vi "AwakeRunnerNoScreen.vi"() -> ()   [LabVIEW 2011]
uses:
  <vilib>/vision/Image Controls.llb/IMAQ Image.ctl
  <vilib>/Instr/_visa.llb/Select Event Type.ctl
  <instrlib>/niHWS/nihws.llb/niHWS Open File Permissions ID.ctl
  <vilib>/DAQmx/read.llb/DAQmx Read (Analog Wfm 1Chan NSamp).vi
  <instrlib>/niHWS/nihws.llb/niHWS Write Analog DBL.vi
  <instrlib>/niHWS/nihws.llb/niHWS Write Analog WDT.vi
  <vilib>/DAQmx/miscellaneous.llb/DAQmx Fill In Error Info.vi
  <vilib>/express/express arith-compare/Formula/XNode/ExpressFormulaBlockNode.xnode
  C:/Program Files/National Instruments/LabVIEW 2011/resource/objmgr/daqmx.rc
  <vilib>/vision/NI_Vision_Development_Module.lvlib
  <vilib>/ptbypt/NI_PtbyPt.lvlib
panel:
  out "Click Value":i8
  out "Image Dst Out":T1
  out "Ephys Rate":dbl=1000.0
  out "Waveform Chart":waveform(dbl)(graph)
  out "Speed History":dbl(graph)
  in  "Magnify":bool
  in  "stop":bool
  out "Camera":T1(plugin-control)
  out "Rec Time":dbl format="%#_3g"
  out "fps":dbl format="%#_2g"
  in  "Rec":bool
  in  "Path":path
  in  "Gain":dbl(slide)=2.6607250597988097 min=1.0 max=3.9810717055349722 scale=0.0..4.0
  in  "Exposure Time":dbl(slide)=16602.0 min=56.0 max=16602.0 scale=0.0..16600.0
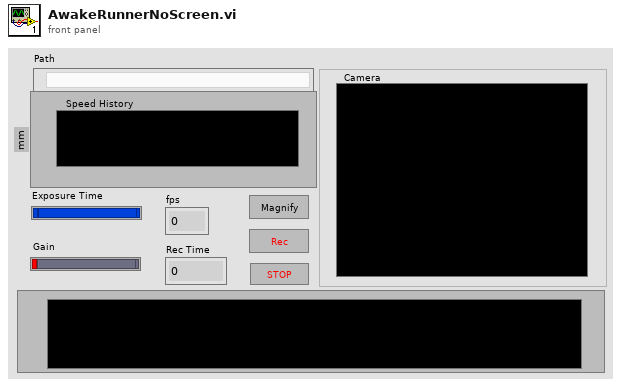
[diagram p1: front panel]
types:
  T1 = typedef "IMAQ Image.ctl" = refnum<image>
  T2 = enum32{"Invalid", "Standard", "Closed", "Hidden", "Minimized", "Maximized"}
  T3 = typedef "niHWS Open File Permissions ID.ctl" = enum32{"Read Only", "Read/Write Existing", "Read/Write/Create New", "Read/Write/Create New Always"}
  T4 = typedef "AviRefnum.ctl" = refnum<k1>
  T5 = typedef "Select Event Type.ctl" = u32
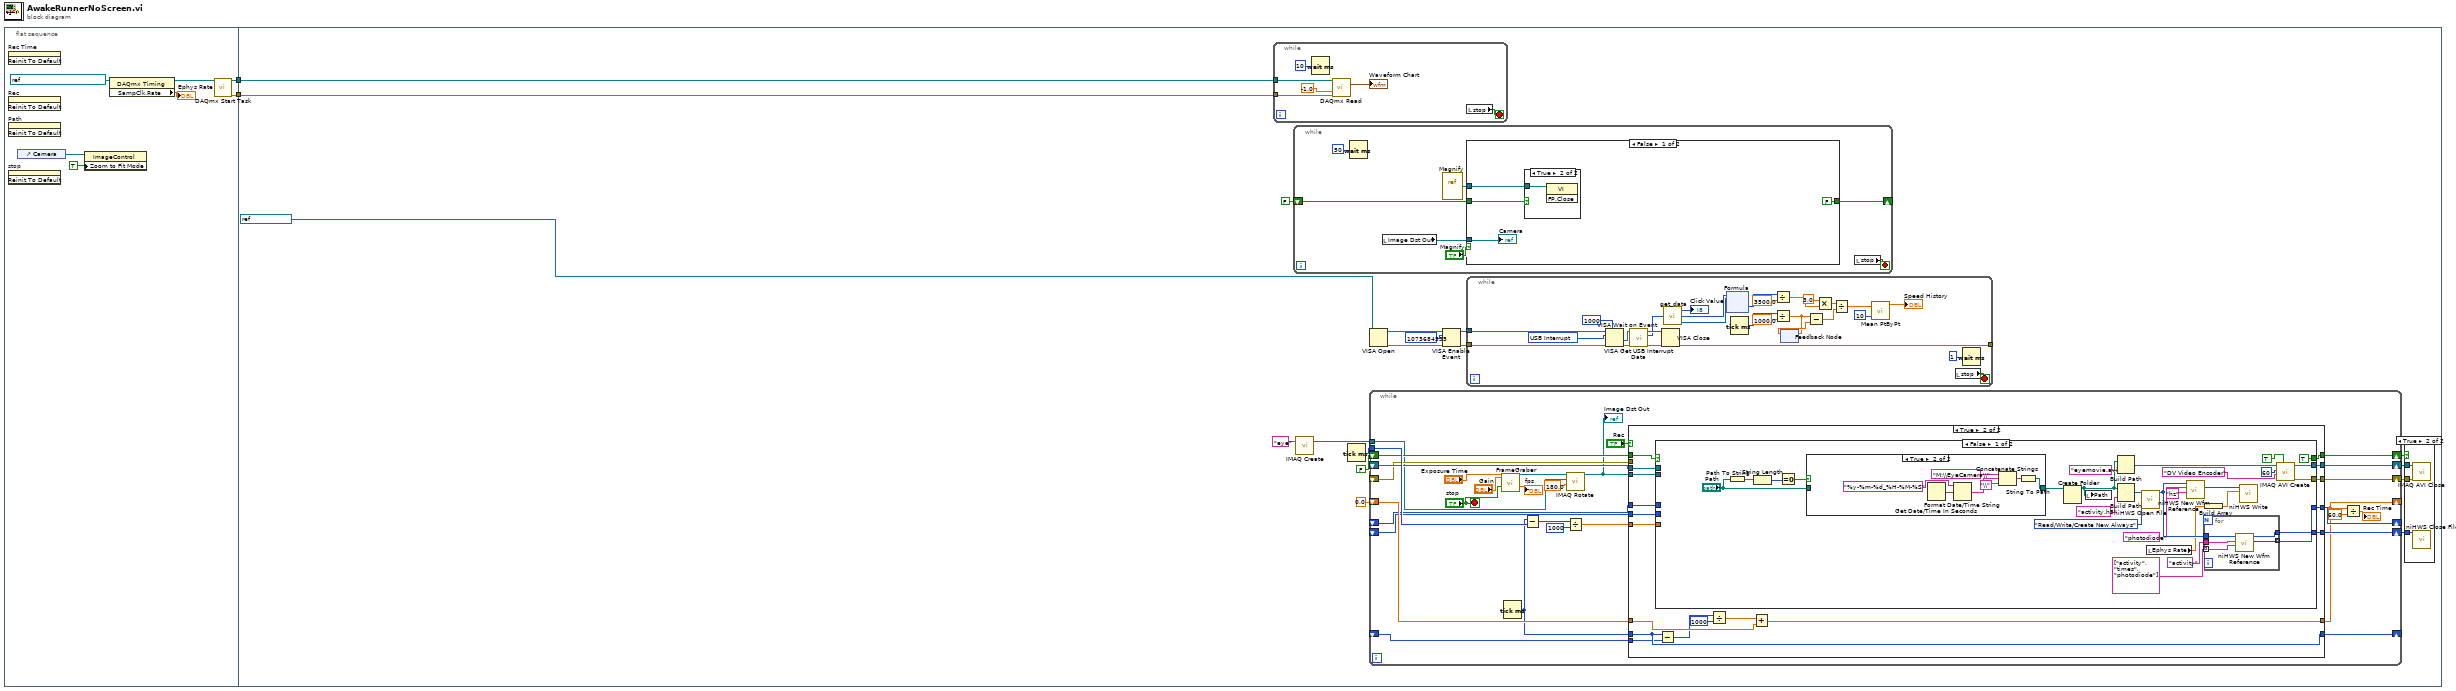
[diagram p0: block diagram]
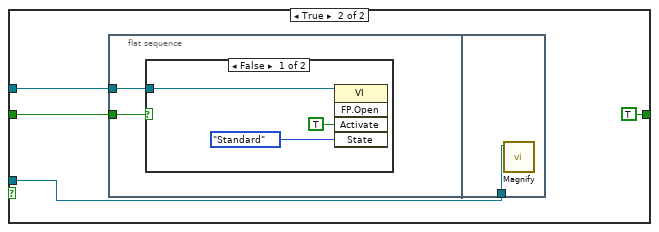
[diagram p3: hidden frame]
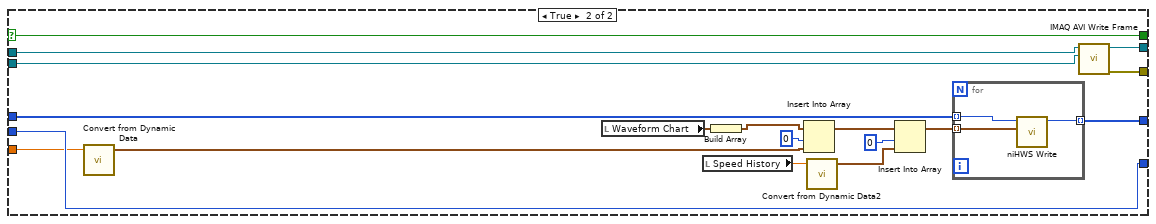
[diagram p8: hidden frame]
diagram:
  n1 = flat-sequence {
    tunnel: [w7] -> w2
    tunnel: [w6] -> w1
    tunnel: w2 -> [w19]
    tunnel: w1 -> [w18]
    frame #0 {
      n2 = invoke on="Rec Time" class="DigNum (strict)" method="Reinit To Default"() -> ()  [unwired: 3 in, 3 out]
      n3 = invoke on="Rec" class="Bool (strict)" method="Reinit To Default"() -> ()  [unwired: 3 in, 3 out]
      n4 = invoke on="Path" class="Path" method="Reinit To Default"() -> ()  [unwired: 3 in, 3 out]
      n5 = invoke on="stop" class="Bool (strict)" method="Reinit To Default"() -> ()  [unwired: 3 in, 3 out]
      n6 = control-ref of="Camera"() -> (w9:refnum<vi>)
      n7 = property on="Property Node" class="ImageControl"(reference=w9, "Zoom to Fit Mode"=TRUE) -> ()  [unwired: 1 in, 2 out]
      n8 = property class="DAQmx Timing"(reference=refnum<k21> "Photodiode Intrinsic Imaging" ("task/channels in")) -> (reference out=w3:refnum<k21>, "SampClk.Rate"=→"Ephys Rate":dbl)  [unwired: 1 in, 1 out]
      n9 = call <vilib>:"DAQmx Start Task.vi"("task/channels in"=w3) -> ("task out"=w7:refnum<k21>, "error out"=w6:errorcluster)  [unwired: 13 in]
    }
    frame #1 {
      n10 = while {
        tunnel: w19 -> [w70]
        tunnel: w18 -> [w69]
        stop <- w71 stop-if-true
        n11 = Wait (ms)(milliseconds to wait=u32 10) -> ()  [unwired: 1 out]
        n12 = call-poly <vilib>:"DAQmx Read.vi"("task/channels in"=w70, "timeout"=-1.0, "error in"=w69) -> ("data"=→"Waveform Chart":waveform(dbl))  [unwired: 10 in, 2 out]
        n13 = local read "stop"() -> (w71:bool)
      }
      n14 = while {
        shift-right: [w75] -> _
        shift-left: FALSE -> [w74]
        stop <- w76 stop-if-true
        n15 = Wait (ms)(milliseconds to wait=u32 50) -> ()  [unwired: 1 out]
        n16 = local read "Image Dst Out"() -> (w72:T1)
        n17 = vi-ref "Magnify.vi"() -> (w78:refnum<vi>)
        n18 = case shown="False" "Magnify" {
          tunnel: w78 -> [w82 w87]
          tunnel: [FALSE TRUE] -> w75
          tunnel: w74 -> [w81 w85]
          tunnel: w72 -> [w79 w84]
          frame False {
            n19 = case shown="True" w81 {
              tunnel: w82 -> [_ w83]
              frame False {
              }
              frame True {
                n20 = invoke class="VI" method="FP.Close"(reference=w83) -> ()  [unwired: 2 in, 3 out]
              }
            }
            "Camera" <- w79
          }
          frame True {
            n21 = flat-sequence {
              tunnel: w87 -> [w89]
              tunnel: w85 -> [w88]
              tunnel: w84 -> [w93]
              frame #0 {
                n22 = case shown="False" w88 {
                  tunnel: w89 -> [w91 _]
                  frame False {
                    n23 = invoke class="VI" method="FP.Open"(reference=w91, "Activate"=TRUE ("Wait Until Done"), "State"=T2."Standard") -> ()  [unwired: 2 in, 5 out]
                  }
                  frame True {
                  }
                }
              }
              frame #1 {
                n24 = call "Magnify.vi"("Camera 2"=w93) -> ()  [unwired: 11 in]
              }
            }
          }
        }
        n25 = local read "stop"() -> (w76:bool)
      }
      n26 = call "IMAQ Create"("Image Name"="eye") -> ("New Image"=w10:T1)  [unwired: 4 in, 1 out]
      n27 = Tick Count (ms)() -> (millisecond timer value=w24:u32)
      n28 = VISA Open(VISA resource name=refnum<visa-resource-name> "Mouse") -> (VISA resource name=w14:refnum<visa-resource-name>, error out=w13:errorcluster)  [unwired: 1 in, 3 out]
      n29 = while {
        tunnel: w24 -> [w125]
        shift-right: [w124] -> _
        shift-left: _ -> [w123]
        shift-right: [w104] -> _
        shift-left: 0.0 -> [w122]
        shift-right: [w112] -> w22
        shift-left: FALSE -> [w113]
        shift-right: [w109] -> _
        shift-left: _ -> [w108]
        shift-right: [w110] -> w21
        shift-left: _ -> [w107]
        shift-right: [w126] -> w27
        shift-left: _ -> [w106]
        shift-right: [w97] -> w26
        shift-left: _ -> [w105]
        tunnel: w10 -> [w98]
        stop <- "stop" stop-if-true
        n30 = call "FrameGraber.vi"("Exposure Time"="Exposure Time", "Gain"="Gain", "Stop (F)"="stop") -> ("Image Out"=w101:T1, "Frame Rate"=→"fps":dbl)  [unwired: 20 in, 3 out]
        n31 = Tick Count (ms)() -> (millisecond timer value=w114:u32)
        n32 = Subtract(x=w114, y=w125) -> (x-y=w117:u32)
        n33 = call "IMAQ Rotate"("Angle (degrees)"=sgl 180.0, "Image Dst"=w98, "Image Src"=w101) -> ("Image Dst Out"=w100:T1)  [unwired: 7 in, 1 out]
        "Image Dst Out" <- w100
        n34 = Divide(x=w117, y=1000) -> (x/y=w115:dbl)
        n35 = case shown="True" "Rec" {
          tunnel: [w128 w142] -> w126
          tunnel: [w127 w141] -> w97
          tunnel: [w132 w148] -> w104
          tunnel: w115 -> [_ w139]
          tunnel: [w133 w151] -> w124
          tunnel: w114 -> [w133 w151]
          tunnel: w123 -> [_ w150]
          tunnel: w122 -> [w132 w149]
          tunnel: w100 -> [_ w140]
          tunnel: w113 -> [w131 w144]
          tunnel: [w131 w143] -> w112
          tunnel: [w129 w138] -> w110
          tunnel: [w130 w137] -> w109
          tunnel: w108 -> [w130 w136]
          tunnel: w107 -> [w129 w135]
          tunnel: w106 -> [w128 w134]
          tunnel: w105 -> [w127 _]
          frame False {
          }
          frame True {
            n36 = case shown="False" w144 {
              selector: w144 -> [_ w209]
              tunnel: [TRUE w209] -> w143
              tunnel: [w175 w208] -> w142
              tunnel: [w174 w207] -> w141
              tunnel: w140 -> [_ w206]
              tunnel: w139 -> [_ w202]
              tunnel: [w159 w205] -> w138
              tunnel: [w158 w194] -> w137
              tunnel: w136 -> [_ w195]
              tunnel: w135 -> [_ w205]
              tunnel: w134 -> [_ w204]
              frame False {
                n37 = Path To String(path="Path") -> (string=w176:string)
                n38 = String Length(string=w176) -> (length=w177:i32)
                n39 = Equal To 0?(x=w177) -> (x = 0?=w165:bool)
                n40 = case shown="True" w165 {
                  tunnel: [w184 w185] -> w163
                  tunnel: "Path" -> [w184 _]
                  frame False {
                  }
                  frame True {
                    n41 = Get Date/Time In Seconds() -> (seconds since 1Jan1904=w191:timestamp)
                    n42 = Format Date/Time String(time format string (%c)="%y-%m-%d_%H-%M-%S", seconds (now)=w191) -> (date/time string=w188:string)  [unwired: 1 in]
                    n43 = Concatenate Strings("M:\\EyeCamera\\", w188, "\\" ("string")) -> (w186:string)
                    n44 = String To Path(string=w186) -> (path=w185:path)
                  }
                }
                n45 = Create Folder(path (use dialog)=w163) -> (created path=w162:path)  [unwired: 2 in, 2 out]
                n46 = local write "Path"(w162) -> ()
                n47 = Build Path(base path=w162, name or relative path="eyemovie.avi" ("search string")) -> (appended path=w168:path)
                n48 = Build Path(base path=w162, name or relative path="activity.h5" ("search string")) -> (appended path=w166:path)
                n49 = call <instrlib>:"niHWS Open File.vi"("permissions (0:read only)"=niHWS_Open_File_Permissions_ID."Read/Write/Create New Always", "file path"=w166) -> ("file handle"=w157:u32)  [unwired: 8 in, 1 out]
                n50 = local read "Ephys Rate"() -> (w153:dbl)
                n51 = call <instrlib>:"niHWS New Wfm Reference.vi"("waveform name (empty)"="hz", "group name (empty)"="photodiode", "file handle in"=w157) -> ("waveform reference"=w154:u32)  [unwired: 6 in, 2 out]
                n52 = for {
                  tunnel: w157 -> [w183]
                  tunnel: [w182] -> w158 mode=indexing
                  tunnel: "activity" ("group name (empty)") -> [w181]
                  tunnel: string[] ["activity", "times", "photodiode"] -> [w180] mode=indexing
                  tunnel: [w179] -> w159
                  n53 = call <instrlib>:"niHWS New Wfm Reference.vi"("waveform name (empty)"=w180, "group name (empty)"=w181, "file handle in"=w183) -> ("waveform reference"=w182:u32, "file handle out"=w179:u32)  [unwired: 6 in, 1 out]
                }
                n54 = Build Array(w153) -> (w152:dbl[])
                n55 = call-poly <instrlib>:"niHWS Write.vi"("data"=w152, "waveform reference in"=w154) -> ()  [unwired: 8 in, 2 out]
                n56 = call "IMAQ AVI Create"("Has Data"=TRUE, "Compression Filter"="DV Video Encoder" ("Compressor"), "Frames Per Second"=u32 60, "AVI Path"=w168) -> ("error out"=w174:errorcluster, "Avi Refnum"=w175:T4)  [unwired: 3 in, 3 out]
              }
              frame True {
                n57 = call "Convert from Dynamic Data"("Dynamic Data Type"=w202) -> ("Waveform"=w201:waveform(dbl))  [unwired: 3 in]
                n58 = local read "Waveform Chart"() -> (w193:waveform(dbl))
                n59 = local read "Speed History"() -> (w198:dbl)
                n60 = Build Array(w193) -> (w192:waveform(dbl)[])
                n61 = Insert Into Array(array=w192, index=0, new element=w201) -> (w199:waveform(dbl)[])
                n62 = call "Convert from Dynamic Data2"("Dynamic Data Type"=w198) -> ("Waveform"=w197:waveform(dbl))  [unwired: 3 in]
                n63 = Insert Into Array(array=w199, index=0, new element=w197) -> (w196:waveform(dbl)[])
                n64 = for {
                  tunnel: w195 -> [w212] mode=indexing
                  tunnel: w196 -> [w211] mode=indexing
                  tunnel: [w210] -> w194 mode=indexing
                  n65 = call-poly <instrlib>:"niHWS Write.vi"("analog waveform"=w211, "waveform reference in"=w212) -> ("waveform reference out"=w210:u32)  [unwired: 8 in, 1 out]
                }
                n66 = call "IMAQ AVI Write Frame"("Image"=w206, "Avi Refnum"=w204) -> ("error out"=w207:errorcluster, "Avi Refnum (duplicate)"=w208:T4)  [unwired: 8 in]
              }
            }
            n67 = Subtract(x=w151, y=w150) -> (x-y=w147:u32)
            n68 = Divide(x=w147, y=1000) -> (x/y=w145:dbl)
            n69 = Add(x=w145, y=w149) -> (x+y=w148:dbl)
          }
        }
        n70 = Divide(x=w104, y=60.0) -> (x/y=→"Rec Time":dbl)
      }
      n71 = VISA Enable Event(8:w13, 10:u32 1073684535 ("event type"), 11:w14) -> (0:w17:errorcluster, 3:w16:refnum<visa-resource-name>)  [unwired: 1 out]
      n72 = while {
        tunnel: w16 -> [w55]
        tunnel: [w54] -> _
        tunnel: w17 -> [w47]
        stop <- w48 stop-if-true
        w46 = T5 1073684535 items=["Service Request"=1073684491, "Trigger"=3221168138, "Clear"=1073684493, "VXI Signal"=1073684512, "VXI/VME Interrupt"=3221168161, "VXI/VME Sysfail"=1073684509, "VXI/VME Sysreset"=1073684510, "GPIB CIC"=1073684498, "GPIB Talk"=1073684499, "GPIB Listen"=1073684500, "PXI Interrupt"=1073684514, "Serial Break"=1073684515, "Serial TermChar"=1073684516, "Serial CTS"=1073684521, "Serial DSR"=1073684522, "Serial DCD"=1073684524, "Serial RI"=1073684526, "Serial Character"=1073684533, "USB Interrupt"=1073684535, "All Enabled"=1073709055] ("Event Type")
        n73 = VISA Wait on Event(7:u32 1000 ("timeout (0)"), 8:w47, 10:w46, 11:w55) -> (0:w51:errorcluster, 1:w50:refnum<visa-resource-name>)  [unwired: 3 out]
        n74 = call <vilib>:"VISA Get USB Interrupt Data.vi"("error in (no error)"=w51, "VISA USB Intr Event"=w50) -> ("error out"=w53:errorcluster, "data buffer"=w44:u8[], "VISA USB Intr Event out"=w52:refnum<visa-resource-name>)  [unwired: 7 out]
        n75 = VISA Close(VISA resource name=w52, error in (no error)=w53) -> (error out=w54:errorcluster)
        n76 = call "get_data.vi"("data buffer"=w44) -> ("Click Value"=→"Click Value":i8, "X Value"=w28:i8, "Y Value"=w29:i8)
        n77 = xnode ("Formula")("X1"=w28, "X2"=w29) -> ("Result"=w41:i8)  [unwired: 1 in, 1 out]
        n78 = Tick Count (ms)() -> (millisecond timer value=w39:u32)
        n79 = Divide(x=w41, y=3500.0 ("DPI")) -> (x/y=w36:dbl)
        n80 = Divide(x=w39, y=1000.0) -> (x/y=w37:dbl)
        n81 = feedback #1() -> (w42:dbl)  [unwired: 1 in]
        n82 = feedback-in #1(w37) -> ()
        n83 = Subtract(x=w37, y=w42) -> (x-y=w40:dbl)
        n84 = Multiply(x=3.0, y=w36) -> (x*y=w35:dbl)
        n85 = Divide(x=w35, y=w40) -> (x/y=w32:dbl)
        n86 = call <vilib>:"Mean PtByPt.vi"("x"=w32, "sample length"=10) -> ("mean"=→"Speed History":dbl)  [unwired: 2 in, 1 out]
        n87 = local read "stop"() -> (w48:bool)
        n88 = Wait (ms)(milliseconds to wait=u32 1) -> ()  [unwired: 1 out]
      }
      n89 = case shown="True" w22 {
        tunnel: w27 -> [_ w96]
        tunnel: w26 -> [_ w95]
        tunnel: w21 -> [_ w94]
        frame False {
        }
        frame True {
          n90 = call "IMAQ AVI Close"("error in (no error)"=w95, "Avi Refnum"=w96) -> ()  [unwired: 9 in, 1 out]
          n91 = call <instrlib>:"niHWS Close File.vi"("file handle"=w94) -> ()  [unwired: 10 in, 1 out]
        }
      }
    }
  }
